vi "Subvi counter U8.vi"(7 "Add?":bool, 9 "Reset":bool) -> (1 "Count":u8)   [LabVIEW 2017]
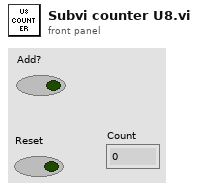
[diagram p1: front panel]
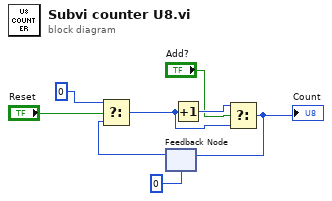
[diagram p0: block diagram]
diagram:
  n1 = feedback #1(u8 0) -> (w2:u8)
  n2 = Select(t=u8 0, s="Reset", f=w2) -> (s? t:f=w4:u8)
  n3 = Increment(x=w4) -> (x+1=w8:u8)
  n4 = Select(t=w8, s="Add?", f=w4) -> (s? t:f=w1:u8)
  "Count" <- w1
  n5 = feedback-in #1(w1) -> ()
